vi "模块一.vi"(8 "ErrorI":errorcluster) -> (0 "ErrorO":errorcluster)   [LabVIEW 2020]
panel:
  in  "Stop":bool
  # "模块1"
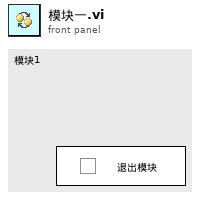
[diagram p1: front panel]
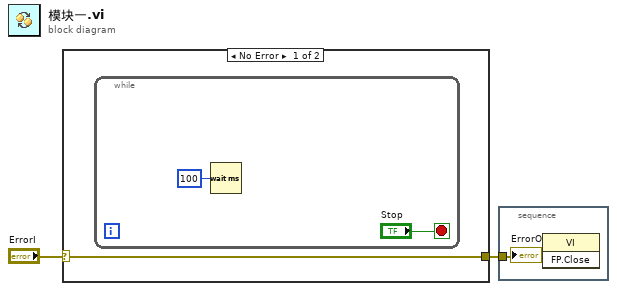
[diagram p0: block diagram]
diagram:
  n1 = case shown="No Error" "ErrorI" {
    selector: "ErrorI" -> [w3 w6]
    tunnel: [w3 w6] -> w1
    frame No Error {
      n2 = while {
        stop <- "Stop" stop-if-true
        n3 = Wait (ms)(milliseconds to wait=u32 100) -> ()  [unwired: 1 out]
      }
    }
    frame Error {
    }
  }
  n4 = stacked-sequence {
    tunnel: w1 -> [w7]
    frame #0 {
      n5 = invoke class="VI" method="FP.Close"() -> ()  [unwired: 3 in, 3 out]
      "ErrorO" <- w7
    }
  }
